vi "Sort_Array_by_1st_col.vi"(1 "2D array to sort":dbl[][](array[numeric]) format="%.2f") -> (0 "Sorted array":dbl[][](array[numeric]) format="%.2f")   [LabVIEW 2016]
doc: "This vi sorts a two-column array in reference to its first column."
panel:
  # "Purpose: This vi sorts a two-column array in reference to its first column."
  # "Instructions: Input a 2D array and then execute the program."
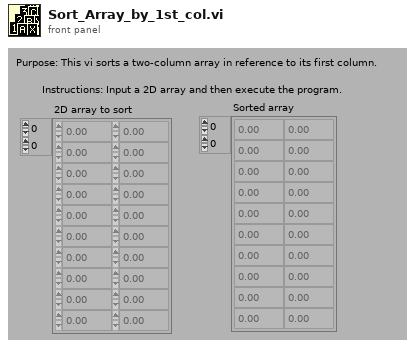
[diagram p1: front panel]
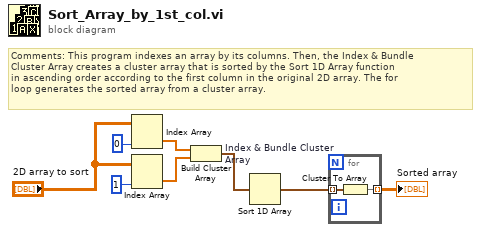
[diagram p0: block diagram]
diagram:
  # "Comments: This program indexes an array by its columns. Then, the Index & Bundle\nCluster Array creates a cluster array that is sorted by the Sort 1D Array function\nin ascending order according to the first column in the original 2D array. The for\nloop generates the sorted array from a cluster array."
  n1 = Index Array(array="2D array to sort", index (col)=0) -> (element=w8:dbl[])  [unwired: 1 in]
  n2 = Index Array(array="2D array to sort", index (col)=1) -> (element=w7:dbl[])  [unwired: 1 in]
  n3 = Build Cluster Array "Index & Bundle Cluster Array"(w8, w7) -> (w6:cluster{dbl, dbl}[])
  n4 = Sort 1D Array(array=w6) -> (sorted array=w5:cluster{dbl, dbl}[])
  n5 = for {
    tunnel: w5 -> [w10] mode=indexing
    tunnel: [w9] -> w4 mode=indexing
    n6 = Cluster To Array(cluster=w10) -> (array=w9:dbl[])
  }
  "Sorted array" <- w4
